vi "removeComments.vi"(3 "Whitespace (\\s\\t\\r\\n)":string="[\\s\\t\\r\\n]+", 4 "Trim Whitespace? (F)":bool, 5 "Comment (#)":string="#", 6 "String":string) -> (0 "Comments":string="header", 1 "Body":string, 2 "Constants":string)   [LabVIEW 2015]
doc: "Removes comments from a string"
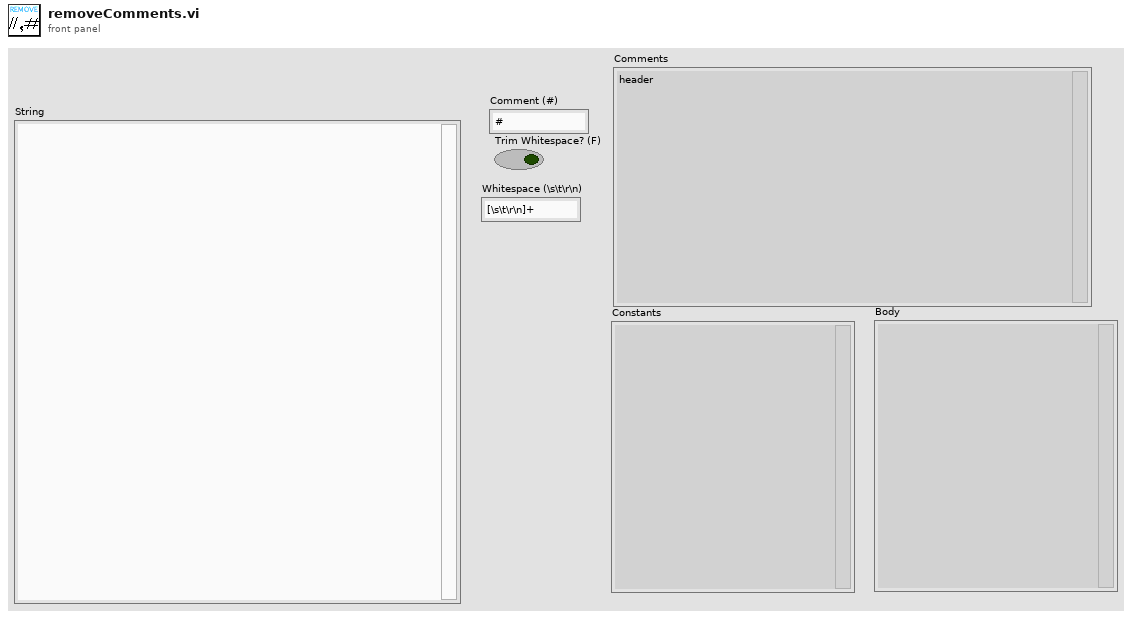
[diagram p1: front panel]
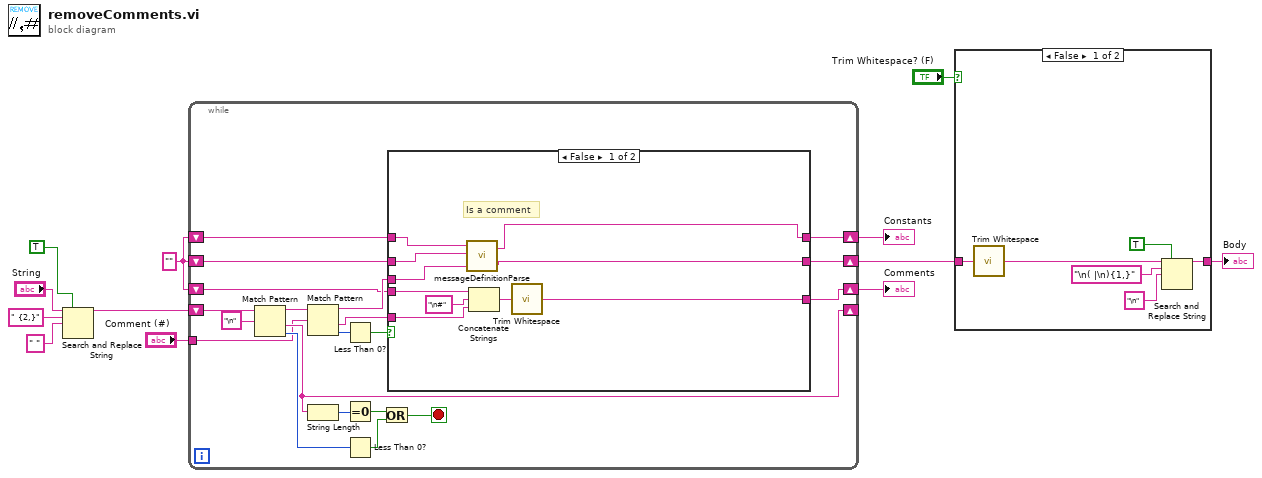
[diagram p0: block diagram]
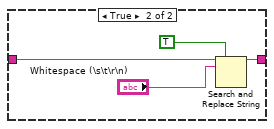
[diagram p2: hidden frame]
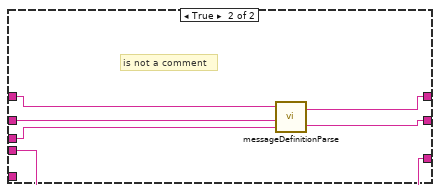
[diagram p3: hidden frame]
diagram:
  w8 = ""
  n1 = Search and Replace String(replace all?=TRUE ("replace all? (F)"), input string="String", search string=" {2,}", replace string=" " ("replace string (\"\")")) -> (result string=w1:string)  [unwired: 4 in, 3 out]
  n2 = while {
    shift-right: [w17] -> w6
    shift-left: w8 -> [w19]
    tunnel: "Comment (#)" -> [w24]
    shift-right: [w25] -> _
    shift-left: w1 -> [w32]
    shift-right: [w16] -> w9
    shift-left: w8 -> [w20]
    shift-right: [w15] -> w7
    shift-left: w8 -> [w21]
    stop <- w26 stop-if-true
    n3 = Match Pattern(string=w32, regular expression="\n") -> (before substring=w18:string, after substring=w25:string, offset past match=w29:i32)  [unwired: 1 in, 1 out]
    n4 = Match Pattern(string=w18, regular expression=w24) -> (before substring=w22:string, after substring=w13:string, offset past match=w14:i32)  [unwired: 1 in, 1 out]
    n5 = String Length(string=w25) -> (length=w30:i32)
    n6 = Less Than 0?(x=w14) -> (x < 0?=w23:bool)
    n7 = Equal To 0?(x=w30) -> (x = 0?=w28:bool)
    n8 = Less Than 0?(x=w29) -> (x < 0?=w27:bool)
    n9 = Or(x=w28, y=w27) -> (x .or. y?=w26:bool)
    n10 = case shown="False" w23 {
      tunnel: w22 -> [w36 w48]
      tunnel: w21 -> [w34 w47]
      tunnel: w20 -> [w37 w46]
      tunnel: w19 -> [w42 w45]
      tunnel: w13 -> [w41 _]
      tunnel: [w39 w45] -> w17
      tunnel: [w35 w44] -> w16
      tunnel: [w33 w43] -> w15
      frame False {
        # "Is a comment"
        n11 = call "messageDefinitionParse.vi"("New String"=w36, "Body"=w37, "Constants"=w34) -> ("Body Out"=w35:string, "Constants Out"=w33:string)
        n12 = Concatenate Strings(w42, "\n#" ("string"), w41) -> (w40:string)
        n13 = call "Trim Whitespace.vi"("string"=w40) -> ("trimmed string"=w39:string)  [unwired: 1 in]
      }
      frame True {
        # "is not a comment"
        n14 = call "messageDefinitionParse.vi"("New String"=w48, "Body"=w46, "Constants"=w47) -> ("Body Out"=w44:string, "Constants Out"=w43:string)
      }
    }
  }
  "Comments" <- w6
  "Constants" <- w7
  n15 = case shown="False" "Trim Whitespace? (F)" {
    tunnel: [w51 w57] -> w12
    tunnel: w9 -> [w54 w55]
    frame False {
      n16 = call "Trim Whitespace.vi"("string"=w54) -> ("trimmed string"=w53:string)  [unwired: 1 in]
      n17 = Search and Replace String(replace all?=TRUE ("replace all? (F)"), input string=w53, search string="\n( |\n){1,}", replace string="\n" ("replace string (\"\")")) -> (result string=w51:string)  [unwired: 4 in, 3 out]
    }
    frame True {
      n18 = Search and Replace String(replace all?=TRUE ("replace all? (F)"), input string=w55, search string="Whitespace (\\s\\t\\r\\n)") -> (result string=w57:string)  [unwired: 5 in, 3 out]
    }
  }
  "Body" <- w12
